vi "Check Range.vi"(7 "Range":T1, 11 "Next Position":T1) -> (3 "In Range Out":bool)   [LabVIEW 2023]
uses:
  Cluster_Point.ctl
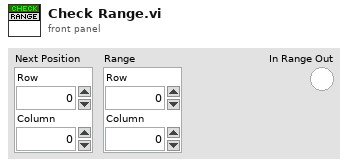
[diagram p1: front panel]
types:
  T1 = typedef "Cluster_Point.ctl" = cluster{"Row":i32, "Column":i32}
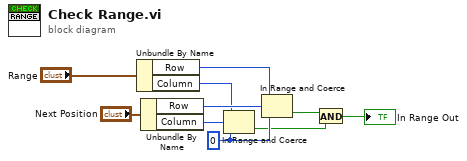
[diagram p0: block diagram]
diagram:
  w8 = 0 ("lower limit")
  n1 = Unbundle By Name("Range") -> ("Row"=w2:i32, "Column"=w1:i32)
  n2 = Unbundle By Name("Next Position") -> ("Row"=w10:i32, "Column"=w7:i32)
  n3 = In Range and Coerce(upper limit=w1, x=w7, lower limit=w8) -> (In Range?=w5:bool)  [unwired: 1 out]
  n4 = In Range and Coerce(upper limit=w2, x=w10, lower limit=w8) -> (In Range?=w6:bool)  [unwired: 1 out]
  n5 = And(x=w6, y=w5) -> (x .and. y?=→"In Range Out":bool)
